vi "GetDLLPath.vi"() -> (0 "DLL Path":path)   [LabVIEW 2023]
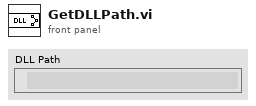
[diagram p1: front panel]
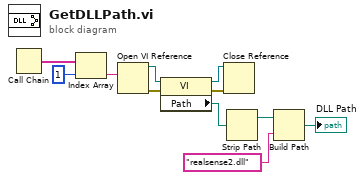
[diagram p0: block diagram]
diagram:
  n1 = Call Chain() -> (call chain=w11:string[])
  n2 = Index Array(array=w11, index=1) -> (element=w10:string)
  n3 = Open VI Reference(vi path=w10) -> (vi reference=w8:refnum<vi>, error out=w4:errorcluster)  [unwired: 5 in]
  n4 = property class="VI"(reference=w8, error in=w4) -> (reference out=w6:refnum<vi>, error out=w5:errorcluster, "Path"=w7:path)
  n5 = Close Reference(reference=w6, error in (no error)=w5) -> ()  [unwired: 1 out]
  n6 = Strip Path(path=w7) -> (stripped path=w3:path)  [unwired: 1 out]
  n7 = Build Path(base path=w3, name or relative path="realsense2.dll") -> (appended path=→"DLL Path":path)
